vi "ConfigurePositionRegulator.vi"(0 "axis in":cluster{"keyHandle":u32, "nodeId":u16}={"keyHandle"=0, "nodeId"=1}, 1 "position gains":T2, 2 "feed forward":T1, 3 "error in (no error)":errorcluster) -> (5 "axis out":cluster{"keyHandle":u32, "nodeId":u16}={"keyHandle"=0, "nodeId"=1}, 7 "error out":errorcluster)   [LabVIEW 2019, in "maxonEPOS.lvlib"]
doc: "<B>ConfigurePositionRegulator</B> writes the position regulation gain and the feed forward parameters to the device."
uses:
  Examples/maxonEPOS.lvlib
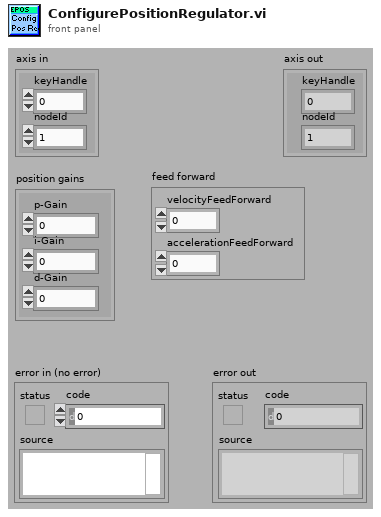
[diagram p1: front panel]
types:
  T1 = cluster{"velocityFeedForward":u16, "accelerationFeedForward":u16}
  T2 = cluster{"p-Gain":u16, "i-Gain":u16, "d-Gain":u16}
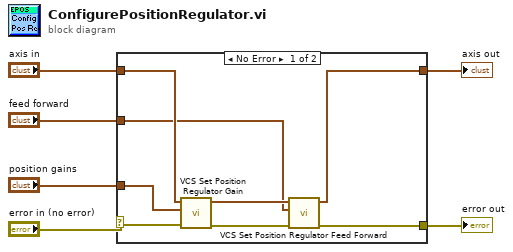
[diagram p0: block diagram]
diagram:
  n1 = case shown="No Error" "error in (no error)" {
    selector: "error in (no error)" -> [w14 w16]
    tunnel: [w10 w16] -> w5
    tunnel: [w9 w15] -> w4
    tunnel: "axis in" -> [w13 w15]
    tunnel: "position gains" -> [w12 _]
    tunnel: "feed forward" -> [w7 _]
    frame No Error {
      n2 = call "VCS Set Position Regulator Gain.vi"("error in (no error)"=w14, "gains"=w12, "axis in"=w13) -> ("error out"=w11:errorcluster, "axis out"=w8:cluster{"keyHandle":u32, "nodeId":u16})  [unwired: 7 in]
      n3 = call "VCS Set Position Regulator Feed Forward.vi"("error in (no error)"=w11, "feed forward"=w7, "axis in"=w8) -> ("error out"=w10:errorcluster, "axis out"=w9:cluster{"keyHandle":u32, "nodeId":u16})  [unwired: 7 in]
    }
    frame Error {
    }
  }
  "error out" <- w5
  "axis out" <- w4
